vi "Validate Report Path.vi"(8 "error in (no error)":errorcluster, 11 "Path":path) -> (0 "error out":errorcluster, 3 "path":path)   [LabVIEW 2020, in "Reports.lvlib" / "Report Generator.lvclass"]
uses:
  Report Generator.lvclass
  Report Generator.lvclass/Report Generator.ctl
  User Interface/Support/Utilities.lvlib
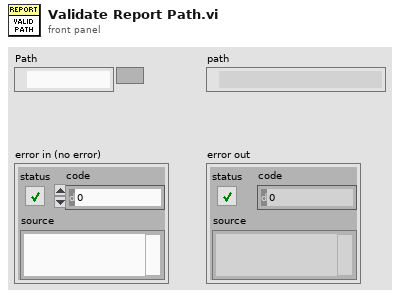
[diagram p1: front panel]
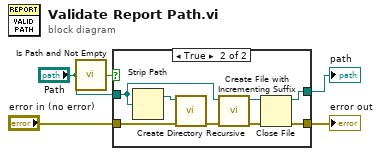
[diagram p0: block diagram]
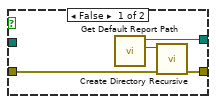
[diagram p2: hidden frame]
diagram:
  n1 = call <vilib>:"Is Path and Not Empty.vi"("path"="Path") -> ("Is Path and Not Empty?"=w3:bool)  [unwired: 4 in]
  n2 = case shown="True" w3 {
    tunnel: "Path" -> [_ w13]
    tunnel: [w9 w17] -> w1
    tunnel: "error in (no error)" -> [w8 w10]
    tunnel: [w7 w16] -> w2
    frame False {
      n3 = call "Get Default Report Path.vi"() -> ("Default Report Directory"=w6:path, "Default Report Path"=w7:path)  [unwired: 10 in]
      n4 = call <vilib>:"Create Directory Recursive.vi"("error in (no error)"=w8, "directory"=w6) -> ("error out"=w9:errorcluster)  [unwired: 3 in, 2 out]
    }
    frame True {
      n5 = Strip Path(path=w13) -> (stripped path=w12:path)  [unwired: 1 out]
      n6 = call <vilib>:"Create Directory Recursive.vi"("error in (no error)"=w10, "directory"=w12) -> ("error out"=w11:errorcluster)  [unwired: 3 in, 2 out]
      n7 = call <vilib>:"Create File with Incrementing Suffix.vi"("error in (no error)"=w11, "file path"=w13) -> ("error out"=w14:errorcluster, "refnum out"=w15:refnum<file>)  [unwired: 7 in, 1 out]
      n8 = Close File(refnum=w15, error in=w14) -> (path=w16:path, error out=w17:errorcluster)
    }
  }
  "error out" <- w1
  "path" <- w2
